vi "16clockpulses one at a time.vi"() -> ()   [LabVIEW 2020]
panel:
  out "SD0":u8[](array[numeric]) format="%.0x"
  out "text":string
  out "Data In":u8[](array[numeric]) format="%.0x"
  out "Batch Length":i32
  out "Actual Bitrate kHz 2":i32=1000
  out "dup Cheetah Handle":i32
  out "Total Shifted Out":i32
  out "Actual Bitrate kHz":i32=1000
  out "error out":errorcluster
  in  "Rds per Sec":dbl=2000.0 max=2000000000.0
  in  "SCLK (kHz)":i32=2000 min=0
  out "Cheetah Handle":i32
  out "SDI":u8[](array[numeric]) format="%.0x"
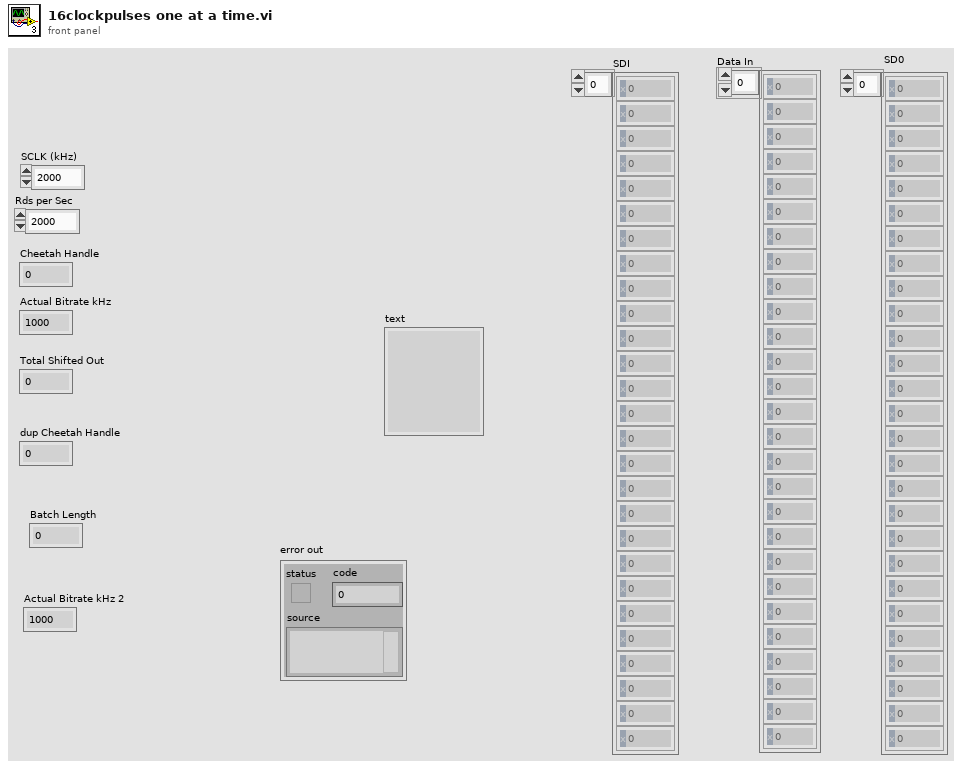
[diagram p1: front panel]
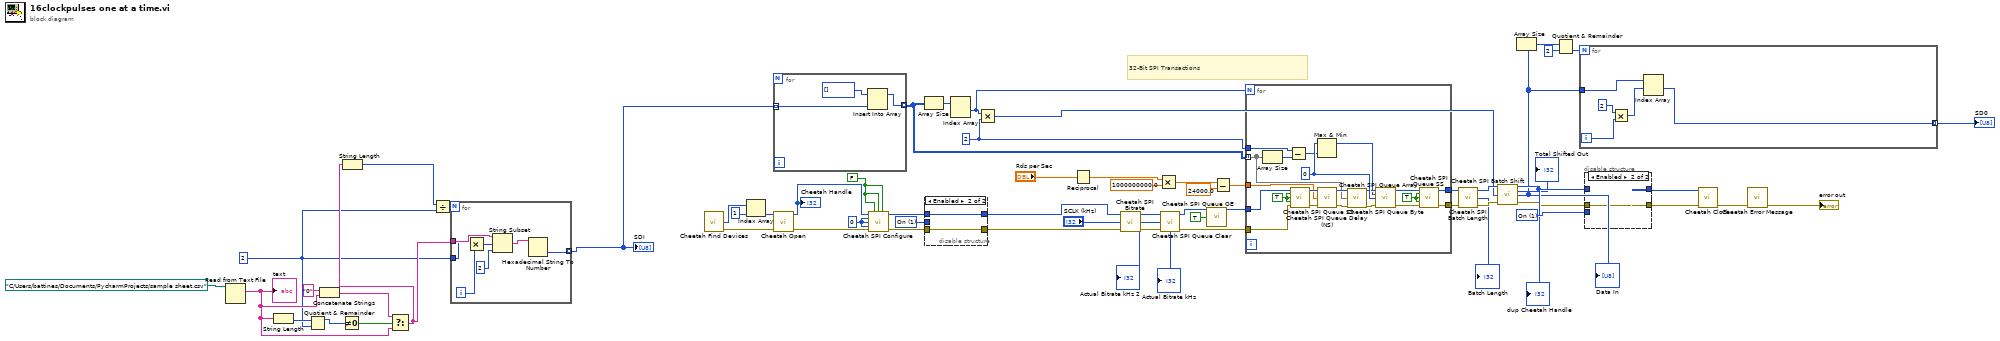
[diagram p0: block diagram]
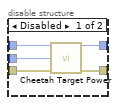
[diagram p2: hidden frame]
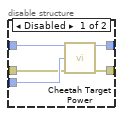
[diagram p3: hidden frame]
diagram:
  w3 = 2 ("x")
  w20 = 2 ("y")
  w42 = u16 1 items=["Off", "On", "Query"] ("Requested Configuration (2: Query)")
  w43 = u16 1 items=["Off", "On", "Query"] ("Requested Configuration (2: Query)")
  w58 = FALSE
  w60 = 0
  # "32-Bit SPI Transactions"
  n1 = Read from Text File(file (use dialog)=path "C:/Users/battines/Documents/PycharmProjects/sample sheet.csv") -> (text=w7:string)  [unwired: 3 in, 3 out]
  "text" <- w7
  n2 = String Length(string=w7) -> (length=w11:i32)
  n3 = Quotient & Remainder(x=w11, y=w3) -> (x-y*floor(x/y)=w10:i32)  [unwired: 1 out]
  n4 = Concatenate Strings("0" ("string"), w7) -> (w8:string)
  n5 = Not Equal To 0?(x=w10) -> (x != 0?=w9:bool)
  n6 = Select(t=w8, s=w9, f=w7) -> (s? t:f=w4:string)
  n7 = String Length(string=w4) -> (length=w5:i32)
  n8 = Divide(x=w5, y=w3) -> (x/y=w6:dbl)
  n9 = for {
    N: w6 -> [_]
    tunnel: w4 -> [w65]
    tunnel: [w66] -> w2 mode=indexing
    tunnel: w3 -> [w64]
    i -> [w68]
    n10 = Multiply(x=w64, y=w68) -> (x*y=w69:i32)
    n11 = String Subset(string=w65, offset (0)=w69, length (rest)=2 ("length (rest)")) -> (substring=w67:string)
    n12 = Hexadecimal String To Number(string=w67) -> (number=w66:u32)  [unwired: 2 in, 1 out]
  }
  "SDI" <- w2
  n13 = call <instrlib>:"Cheetah Find Devices.vi"() -> ("Ports"=w61:u16[], "error out"=w57:errorcluster)  [unwired: 13 in, 1 out]
  n14 = Index Array(array=w61, index=1) -> (element=w49:u16)
  n15 = for {
    tunnel: [w72] -> w29 mode=indexing
    tunnel: w2 -> [w70] mode=indexing
    n16 = Insert Into Array(array=u8[] [], new element=w70) -> (w72:u8[])  [unwired: 1 in]
  }
  n17 = call <instrlib>:"Cheetah Open.vi"("Port Number (0)"=w49, "error in (no error)"=w57) -> ("Cheetah Handle"=w54:i32, "error out"=w56:errorcluster)  [unwired: 12 in]
  "Cheetah Handle" <- w54
  n18 = call <instrlib>:"Cheetah SPI Configure.vi"("Cheetah Handle"=w54, "SS0 Active High? (False)"=w58, "SS1 Active High? (False)"=w58, "SS2 Active High? (False)"=w58, "Polarity (0: Rising/Falling)"=w60, "Phase (0: Sample/Setup)"=w60, "Bitorder (0: MSB)"=w60, "error in (no error)"=w56) -> ("dup Cheetah Handle"=w53:i32, "error out"=w55:errorcluster)  [unwired: 6 in]
  n19 = Array Size(array=w29) -> (size(s)=w41:i32[])
  n20 = disable-structure shown="Enabled" {
    disable-tunnel: w55 -> [w77 w78]
    disable-tunnel: w53 -> [w76 w79]
    disable-tunnel: [w75 w78] -> w52
    disable-tunnel: [w74 w79] -> w50
    disable-tunnel: w42 -> [w73 _]
    frame Disabled {
      n21 = call <instrlib>:"Cheetah Target Power.vi"("Cheetah Handle"=w76, "Requested Configuration (2: Query)"=w73, "error in (no error)"=w77) -> ("dup Cheetah Handle"=w74:i32, "error out"=w75:errorcluster)  [unwired: 10 in, 1 out]
    }
    frame Enabled {
    }
  }
  n22 = Index Array(array=w41) -> (element #1=w16:i32)  [unwired: 2 in, 1 out]
  n23 = Multiply(x=w16, y=w20) -> (x*y=w15:i32)
  n24 = Reciprocal(x="Rds per Sec") -> (1/x=w22:dbl)
  n25 = call <instrlib>:"Cheetah SPI Bitrate.vi"("Cheetah Handle"=w50, "Requested Bitrate kHz (1000)"="SCLK (kHz)", "error in (no error)"=w52) -> ("dup Cheetah Handle"=w48:i32, "Actual Bitrate kHz"=→"Actual Bitrate kHz" →"Actual Bitrate kHz 2":i32, "error out"=w47:errorcluster)  [unwired: 10 in]
  n26 = Multiply(x=w22, y=1000000000.0) -> (x*y=w25:dbl)
  n27 = call <instrlib>:"Cheetah SPI Queue Clear.vi"("Cheetah Handle"=w48, "error in (no error)"=w47) -> ("dup Cheetah Handle"=w40:i32, "error out"=w59:errorcluster)  [unwired: 12 in]
  n28 = call <instrlib>:"Cheetah SPI Queue OE.vi"("Cheetah Handle"=w40, "Output Enable (on)"=TRUE) -> ("dup Cheetah Handle"=w39:i32)  [unwired: 12 in, 1 out]
  n29 = Subtract(x=w25, y=24000.0) -> (x-y=w23:dbl)
  n30 = for {
    N: w16 -> [_]
    tunnel: w59 -> [w86]
    tunnel: w39 -> [w87]
    tunnel: w29 -> [w88] mode=indexing
    tunnel: [w85] -> w37
    tunnel: [w84] -> w36
    tunnel: w23 -> [w81]
    tunnel: w20 -> [w82]
    w92 = TRUE
    w95 = 0
    w83 = TRUE
    n31 = Array Size(array=w88) -> (size(s)=w89:i32)
    n32 = Subtract(x=w82, y=w89) -> (x-y=w93:i32)
    n33 = call <instrlib>:"Cheetah SPI Queue SS.vi"("Cheetah Handle"=w87, "SS0 Assert? (True)"=w83, "SS1 Assert? (True)"=w83, "SS2 Assert? (True)"=w83, "error in (no error)"=w86) -> ("dup Cheetah Handle"=w100:i32, "error out"=w99:errorcluster)  [unwired: 9 in]
    n34 = Max & Min(x=w95, y=w93) -> (max(x,y)=w80:i32)  [unwired: 1 out]
    n35 = call <instrlib>:"Cheetah SPI Queue Delay (NS).vi"("Cheetah Handle"=w100, "Delay NS (1000)"=w81, "error in (no error)"=w99) -> ("dup Cheetah Handle"=w98:i32, "error out"=w97:errorcluster)  [unwired: 10 in, 1 out]
    n36 = call <instrlib>:"Cheetah SPI Queue Array.vi"("Cheetah Handle"=w98, "Data Out (none)"=w88, "error in (no error)"=w97) -> ("dup Cheetah Handle"=w94:i32, "error out"=w96:errorcluster)  [unwired: 11 in]
    n37 = call <instrlib>:"Cheetah SPI Queue Byte.vi"("Cheetah Handle"=w94, "Byte Count (1)"=w80, "Byte Value (0x00)"=w95, "error in (no error)"=w96) -> ("dup Cheetah Handle"=w91:i32, "error out"=w90:errorcluster)  [unwired: 10 in]
    n38 = call <instrlib>:"Cheetah SPI Queue SS.vi"("Cheetah Handle"=w91, "SS0 Assert? (True)"=w92, "SS1 Assert? (True)"=w92, "SS2 Assert? (True)"=w92, "error in (no error)"=w90) -> ("dup Cheetah Handle"=w84:i32, "error out"=w85:errorcluster)  [unwired: 9 in]
  }
  n39 = call <instrlib>:"Cheetah SPI Batch Length.vi"("Cheetah Handle"=w36, "error in (no error)"=w37) -> ("dup Cheetah Handle"=w35:i32, "Batch Length"=→"Batch Length":i32, "error out"=w34:errorcluster)  [unwired: 11 in]
  n40 = call <instrlib>:"Cheetah SPI Batch Shift.vi"("Cheetah Handle"=w35, "Max Bytes to Retrieve (256)"=w15, "error in (no error)"=w34) -> ("dup Cheetah Handle"=w33:i32, "Total Shifted Out"=→"Total Shifted Out":i32, "Data In"=w17:u8[], "error out"=w28:errorcluster)  [unwired: 9 in]
  "dup Cheetah Handle" <- w33
  "Data In" <- w17
  n41 = Array Size(array=w17) -> (size(s)=w32:i32)
  n42 = Quotient & Remainder(x=w32, y=2) -> (floor(x/y)=w30:i32)  [unwired: 1 out]
  n43 = for {
    N: w30 -> [_]
    tunnel: w17 -> [w104]
    tunnel: [w105] -> _ mode=indexing
    tunnel: [w105] -> w1 mode=indexing
    i -> [w102]
    n44 = Multiply(x=2, y=w102) -> (x*y=w101:i32)
    n45 = Index Array(array=w104, index #1=w101) -> (element #1=w105:u8)  [unwired: 1 in, 1 out]
  }
  "SD0" <- w1
  n46 = disable-structure shown="Enabled" {
    disable-tunnel: [w110 _] -> w46
    disable-tunnel: [w109 w111] -> w45
    disable-tunnel: w43 -> [w108 _]
    disable-tunnel: w33 -> [w107 _]
    disable-tunnel: w28 -> [w106 w111]
    frame Disabled {
      n47 = call <instrlib>:"Cheetah Target Power.vi"("Cheetah Handle"=w107, "Requested Configuration (2: Query)"=w108, "error in (no error)"=w106) -> ("dup Cheetah Handle"=w110:i32, "error out"=w109:errorcluster)  [unwired: 10 in, 1 out]
    }
    frame Enabled {
    }
  }
  n48 = call <instrlib>:"Cheetah Close.vi"("Cheetah Handle"=w46, "error in (no error)"=w45) -> ("error out"=w44:errorcluster)  [unwired: 12 in, 1 out]
  n49 = call <instrlib>:"Cheetah Error Message.vi"("error in (no error)"=w44) -> ("error out"=→"error out":errorcluster)  [unwired: 10 in, 4 out]
